vi "Safe.vi"() -> ()   [LabVIEW 2016]
uses:
  VIs/Control/SafeControl.ctl
panel:
  in  "Command":string
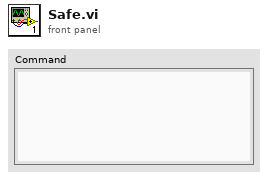
[diagram p1: front panel]
types:
  T1 = typedef "SafeControl.ctl" = enum16{"Idle", "Abort", "Initialize", "BeforeExcute"}
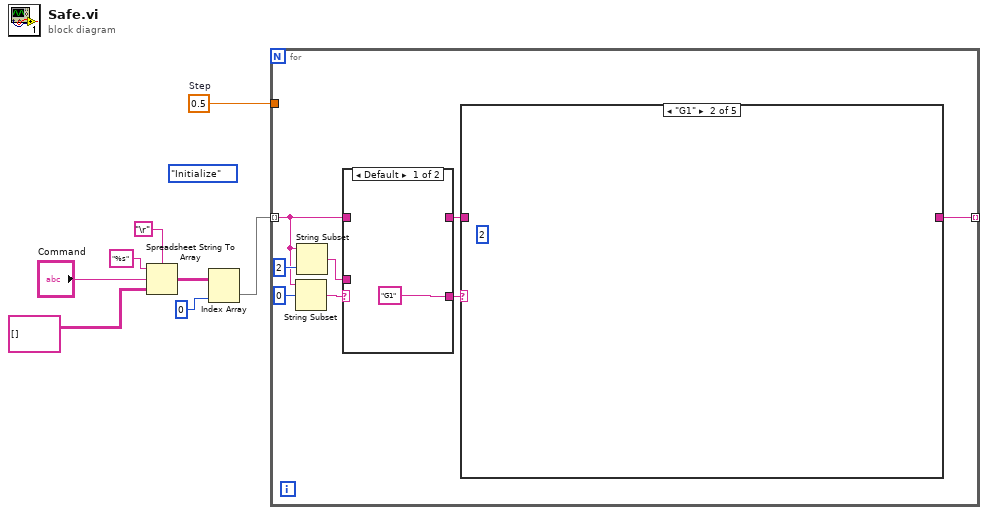
[diagram p0: block diagram]
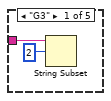
[diagram p3: hidden frame]
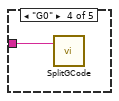
[diagram p5: hidden frame]
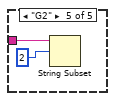
[diagram p6: hidden frame]
diagram:
  w1 = 0.5  # Step
  (unwired) SafeControl."Initialize"
  n1 = Spreadsheet String To Array(delimiter (Tab)="\r", format string="%s", spreadsheet string="Command", array type (2D Dbl)=string[][] []) -> (array=w4:string[][])
  n2 = Index Array(array=w4, index (col)=0) -> (element=w2:string[])  [unwired: 1 in]
  n3 = for {
    tunnel: w2 -> [w10] mode=indexing
    tunnel: [w11] -> _ mode=indexing
    tunnel: w1 -> [_]
    n4 = String Subset(string=w10, offset (0)=0) -> (substring=w15:string)  [unwired: 1 in]
    n5 = String Subset(string=w10, length (rest)=2) -> (substring=w13:string)  [unwired: 1 in]
    n6 = case shown="Default" w15 {
      tunnel: ["G1" w18] -> w12
      tunnel: w13 -> [_ w18]
      tunnel: w10 -> [_ _]
      tunnel: [_ _] -> w9
      frame Default {
      }
      frame "G" {
      }
    }
    n7 = case shown="\"G1\"" w12 {
      tunnel: w9 -> [w19 w21 w22 w23 w24]
      tunnel: [_ _ w22 _ _] -> w11
      frame "G3" {
        n8 = String Subset(string=w19, offset (0)=2) -> ()  [unwired: 1 in, 1 out]
      }
      frame "G1" {
        (unwired) 2
      }
      frame Default {
      }
      frame "G0" {
        n9 = call "SplitGCode.vi"("string"=w23) -> ()  [unwired: 1 in, 2 out]
      }
      frame "G2" {
        n10 = String Subset(string=w24, offset (0)=2) -> ()  [unwired: 1 in, 1 out]
      }
    }
  }
